vi "WriteMicroseconds.vi"(8 "error in (no error)":errorcluster, 9 "Microsec":u16, 10 "Led num":u8, 11 "PCA in":refnum<class "PCA.lvclass">) -> (0 "error out":errorcluster, 3 "PCA out":refnum<class "PCA.lvclass">)   [LabVIEW 2022 SP3, in "PCA9685.lvlib" / "PCA.lvclass"]
uses:
  PCA.lvclass
  PCA.lvclass/PCA.ctl
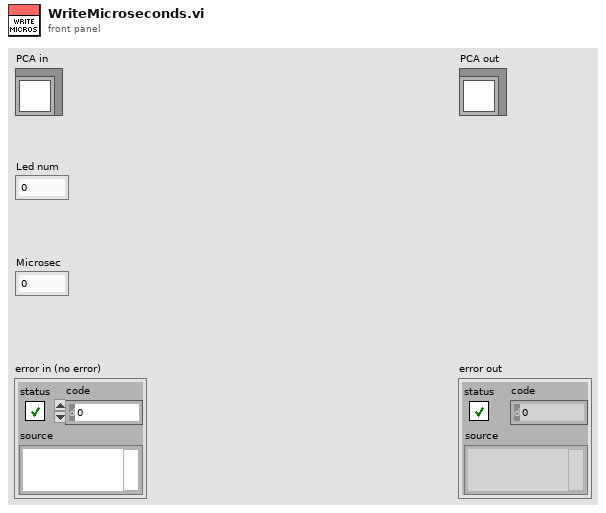
[diagram p1: front panel]
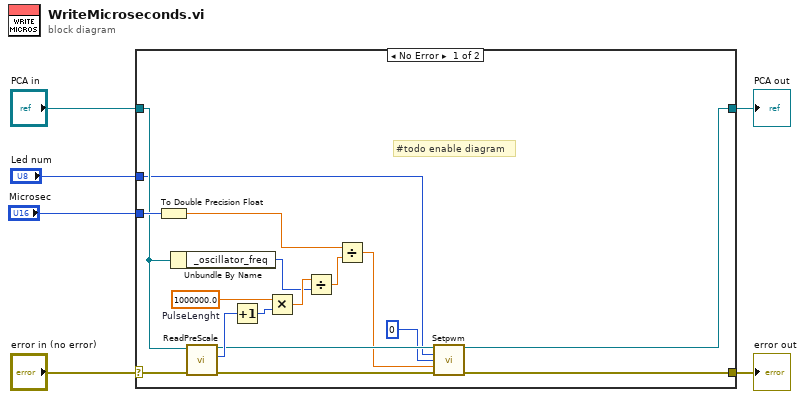
[diagram p0: block diagram]
diagram:
  n1 = case shown="No Error" "error in (no error)" {
    selector: "error in (no error)" -> [w22 w25]
    tunnel: [w12 w25] -> w5
    tunnel: [w7 w24] -> w3
    tunnel: "PCA in" -> [w18 w24]
    tunnel: "Microsec" -> [w23 _]
    tunnel: "Led num" -> [w10 _]
    frame No Error {
      w19 = 1000000.0  # PulseLenght
      # "#todo enable diagram"
      n2 = To Double Precision Float(number=w23) -> (double precision float=w14:dbl)
      n3 = Unbundle By Name(w18) -> ("_oscillator_freq"=w16:u32)
      n4 = call "ReadPreScale.vi"("error in (no error)"=w22, "PCA in"=w18) -> ("error out"=w13:errorcluster, "Prescale"=w21:u8, "PCA out"=w11:refnum<class "PCA.lvclass">)  [unwired: 7 in]
      n5 = Increment(x=w21) -> (x+1=w20:u8)
      n6 = Multiply(x=w19, y=w20) -> (x*y=w17:dbl)
      n7 = Divide(x=w17, y=w16) -> (x/y=w15:dbl)
      n8 = Divide(x=w14, y=w15) -> (x/y=w9:dbl)
      n9 = call "Setpwm.vi"("PCA in"=w11, "Led num"=w10, "on"=0, "off"=w9, "error in (no error)"=w13) -> ("PCA out"=w7:refnum<class "PCA.lvclass">, "error out"=w12:errorcluster)  [unwired: 8 in, 1 out]
    }
    frame Error {
    }
  }
  "error out" <- w5
  "PCA out" <- w3
